vi "Prepare Recording Settings.vi"(8 "error in":errorcluster, 11 "measurement configuration in":T2={"Resource Name(s)"=[], "Number Of Records"=2, "Timeout (s)"=5.0, "Configuration File Path"="", "Delay Mode"="On", "Trigger Position"=0.0, "Length Unit"="Percentage", "Record Length"=100.0, "Stream To File Path"=""} {"Record Length" format="%#_6ps"; "Trigger Position" min=0.0 max=100.0 step=5.0 format="%#_6ps"; "Timeout (s)" format="%#_6p"}) -> (0 "error out":errorcluster, 2 "Recording Settings":T1={"Number of Records"=0, "Plot Names"=[], "Stream To File?"=FALSE, "TDMS Session"=refnum, "Fetch Timeout"=0.0, "Channels Per Record"=1} {"Fetch Timeout" format="%.2f"}, 3 "measurement configuration out":T2={"Resource Name(s)"=[], "Number Of Records"=2, "Timeout (s)"=5.0, "Configuration File Path"="", "Delay Mode"="On", "Trigger Position"=0.0, "Length Unit"="Percentage", "Record Length"=100.0, "Stream To File Path"=""} {"Record Length" format="%#_6ps"; "Trigger Position" min=0.0 max=100.0 step=5.0 format="%#_6ps"; "Timeout (s)" format="%#_6p"})   [LabVIEW 2025, in "Ni-Scope-Multirecords.lvclass"]
uses:
  Ni-Scope-Multirecords.lvclass
  Measurement Configuration.ctl
  Recording Settings.ctl
  <vilib>/Utility/error.llb/Error Cluster From Error Code.vi
  <vilib>/ErrorRing/Error Ring.xnode
  Ni-Scope-Multirecords.lvclass/Ni-Scope-Multirecords.ctl
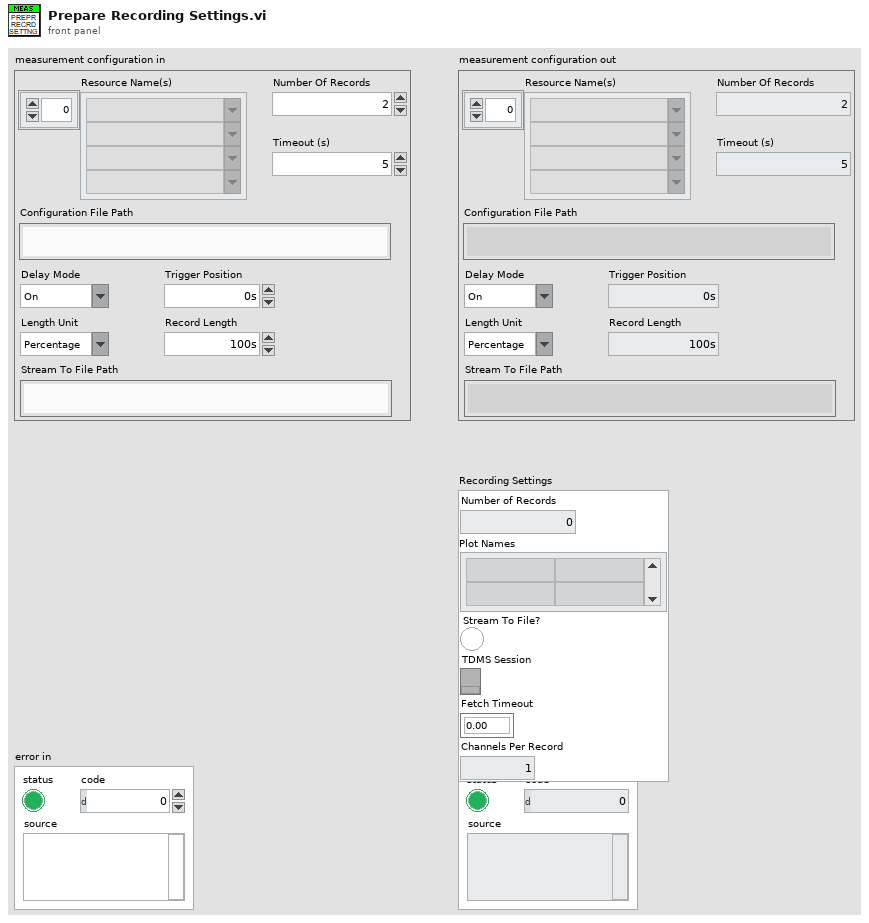
[diagram p1: front panel]
types:
  T1 = typedef "Ni-Scope-Multirecords.lvclass/Recording Settings.ctl" = cluster{"Number of Records":i32, "Plot Names":string[][], "Stream To File?":bool, "TDMS Session":refnum<k34>, "Fetch Timeout":dbl, "Channels Per Record":i32}
  T2 = typedef "Ni-Scope-Multirecords.lvclass/Measurement Configuration.ctl" = cluster{"Resource Name(s)":string[], "Number Of Records":i32, "Timeout (s)":dbl, "Configuration File Path":string, "Delay Mode":string, "Trigger Position":dbl, "Length Unit":string, "Record Length":dbl, "Stream To File Path":string}
  T3 = enum16{"open", "open or create", "create or replace", "create", "open (read-only)"}
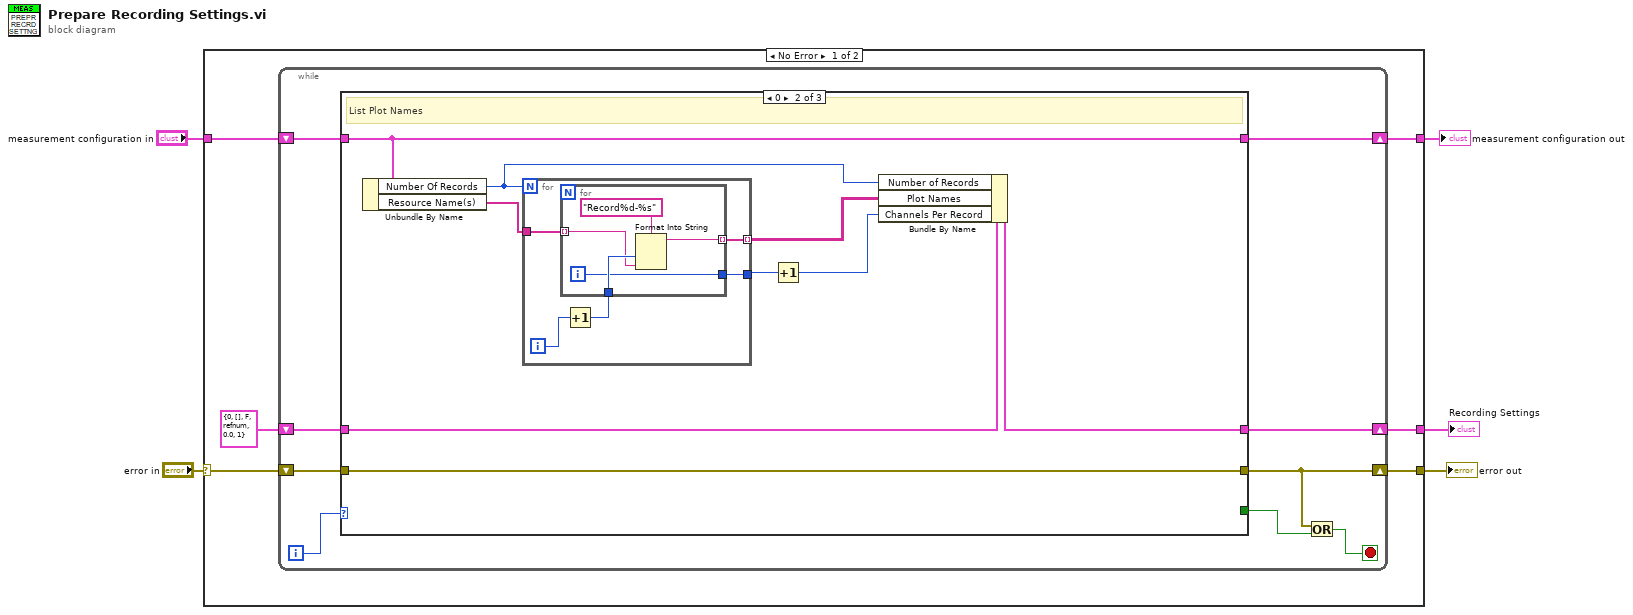
[diagram p0: block diagram]
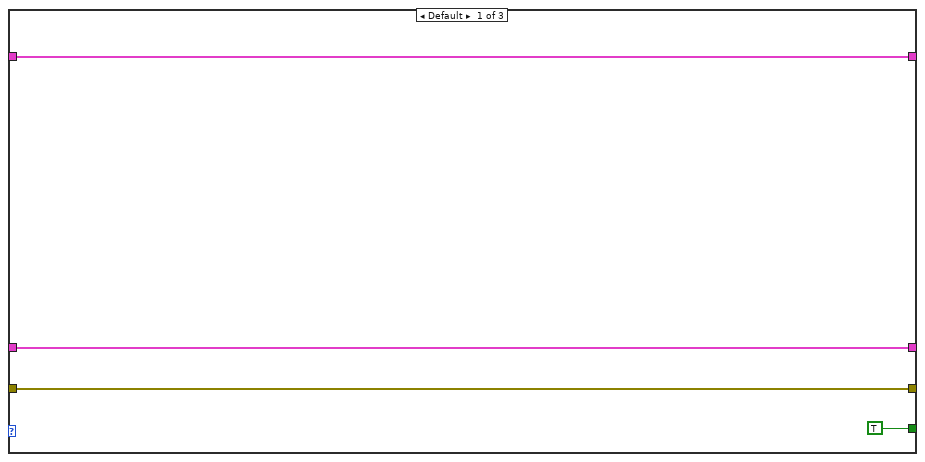
[diagram p2: hidden frame]
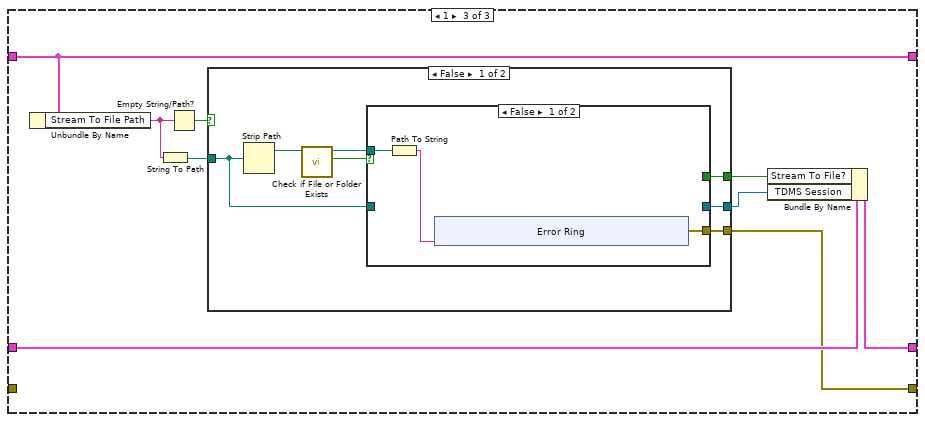
[diagram p3: hidden frame]
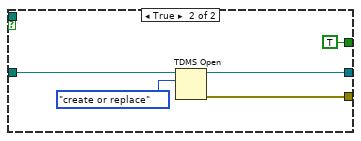
[diagram p4: hidden frame]
diagram:
  n1 = case shown="No Error" "error in" {
    selector: "error in" -> [w11 w75]
    tunnel: "measurement configuration in" -> [w10 w76]
    tunnel: [w9 w76] -> w3
    tunnel: [w8 w75] -> w2
    tunnel: [w6 _] -> w1
    frame No Error {
      n2 = while {
        shift-right: [w16] -> w8
        shift-left: w11 -> [w19]
        shift-right: [w17] -> w9
        shift-left: w10 -> [w18]
        shift-right: [w12] -> w6
        shift-left: T1 {"Number of Records"=0, "Plot Names"=[], "Stream To File?"=FALSE, "TDMS Session"=refnum, "Fetch Timeout"=0.0, "Channels Per Record"=1} ("Recording Settings") -> [w14]
        i -> [w20]
        stop <- w15 stop-if-true
        n3 = case shown="0" w20 {
          tunnel: w19 -> [w24 w33 _]
          tunnel: [w24 w33 w44] -> w16
          tunnel: w18 -> [w23 w32 w52]
          tunnel: [w23 w32 w52] -> w17
          tunnel: [TRUE _ _] -> w13
          tunnel: [w21 w29 w47] -> w12
          tunnel: w14 -> [w21 w30 w48]
          frame Default {
          }
          frame 0 {
            # "List Plot Names"
            n4 = Unbundle By Name(w32) -> ("Number Of Records"=w28:i32, "Resource Name(s)"=w31:string[])
            n5 = for {
              N: w28 -> [_]
              tunnel: w31 -> [w36]
              tunnel: [w35] -> w27 mode=indexing
              tunnel: [w34] -> w26
              i -> [w38]
              n6 = Increment(x=w38) -> (x+1=w37:i32)
              n7 = for {
                tunnel: w37 -> [w42]
                tunnel: w36 -> [w41] mode=indexing
                tunnel: [w40] -> w35 mode=indexing
                tunnel: [w39] -> w34
                i -> [w39]
                n8 = Format Into String(format string="Record%d-%s", w42, w41) -> (resulting string=w40:string)  [unwired: 2 in, 1 out]
              }
            }
            n9 = Increment(x=w26) -> (x+1=w25:i32)
            n10 = Bundle By Name(cluster=w30, "Number of Records"=w28, "Plot Names"=w27, "Channels Per Record"=w25) -> (w29:T1)
          }
          frame 1 {
            n11 = Unbundle By Name(w52) -> ("Stream To File Path"=w51:string)
            n12 = String To Path(string=w51) -> (path=w50:path)
            n13 = Empty String/Path?(string/path=w51) -> (empty?=w49:bool)
            n14 = case shown="False" w49 {
              tunnel: w50 -> [w57 _]
              tunnel: [w55 _] -> w46
              tunnel: [w54 _] -> w45
              tunnel: [w53 _] -> w44
              frame False {
                n15 = Strip Path(path=w57) -> (stripped path=w59:path)  [unwired: 1 out]
                n16 = call <vilib>:"Check if File or Folder Exists.vi"("path"=w59) -> ("file or folder exists?"=w58:bool, "dup path"=w56:path)  [unwired: 8 in, 1 out]
                n17 = case shown="False" w58 {
                  tunnel: w57 -> [_ w73]
                  tunnel: w56 -> [w62 _]
                  tunnel: [w60 w72] -> w53
                  tunnel: [_ TRUE] -> w55
                  tunnel: [_ w70] -> w54
                  frame False {
                    n18 = Path To String(path=w62) -> (string=w61:string)
                    n19 = xnode "Error Ring"("parameter 0"=w61) -> ("error out"=w60:errorcluster)
                  }
                  frame True {
                    n20 = TDMS Open(10:T3."create or replace" ("operation (0:open)"), 11:w73) -> (0:w72:errorcluster, 3:w70:refnum<k34>)  [unwired: 5 in]
                  }
                }
              }
              frame True {
                # "Stream to file path not specified. No need to stream."
              }
            }
            n21 = Bundle By Name(cluster=w48, "Stream To File?"=w46, "TDMS Session"=w45) -> (w47:T1)
          }
        }
        n22 = Or(x=w16, y=w13) -> (x .or. y?=w15:bool)
      }
    }
    frame Error {
    }
  }
  "measurement configuration out" <- w3
  "error out" <- w2
  "Recording Settings" <- w1
